vi "getFocus.vi"(5 "img":u32, 7 "imgLineWidth":i32, 8 "error in (no error)":errorcluster, 9 "interactive":i32, 10 "imgHeight":i32, 11 "imgWidth":i32) -> (0 "error out":errorcluster, 2 "focus":sgl, 3 "return value":i32)   [LabVIEW 2011, in "gVision.lvlib"]
uses:
  gVision.lvlib
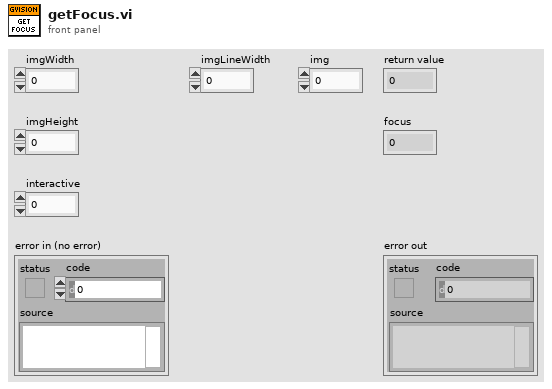
[diagram p1: front panel]
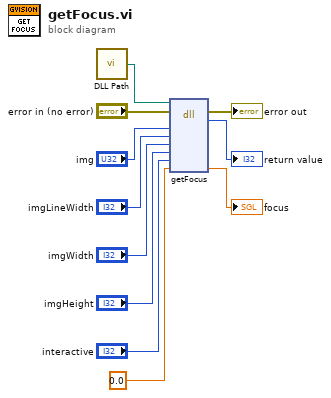
[diagram p0: block diagram]
diagram:
  n1 = call "DLL Path.vi"() -> ("DLL Path"=w1:path)  [unwired: 5 in]
  n2 = dll-call lib="?" fn="getFocus"(path in=w1, error in="error in (no error)", "img"="img", "imgLineWidth"="imgLineWidth", "imgWidth"="imgWidth", "imgHeight"="imgHeight", "interactive"="interactive", "focus"=sgl 0.0) -> (error out=→"error out":errorcluster, "return type"=→"return value":i32, "focus"=→"focus":sgl)  [unwired: 6 in, 1 out]
